vi "auton safty.vi"(11 "Updated Drive Metrics in":T1) -> (3 "Updated Drive Metrics out":T1)   [LabVIEW 2014]
uses:
  Lightning base/Drive Train Metrics.ctl
  Lightning base/CmdFlag.ctl
  Robot Global Data.vi
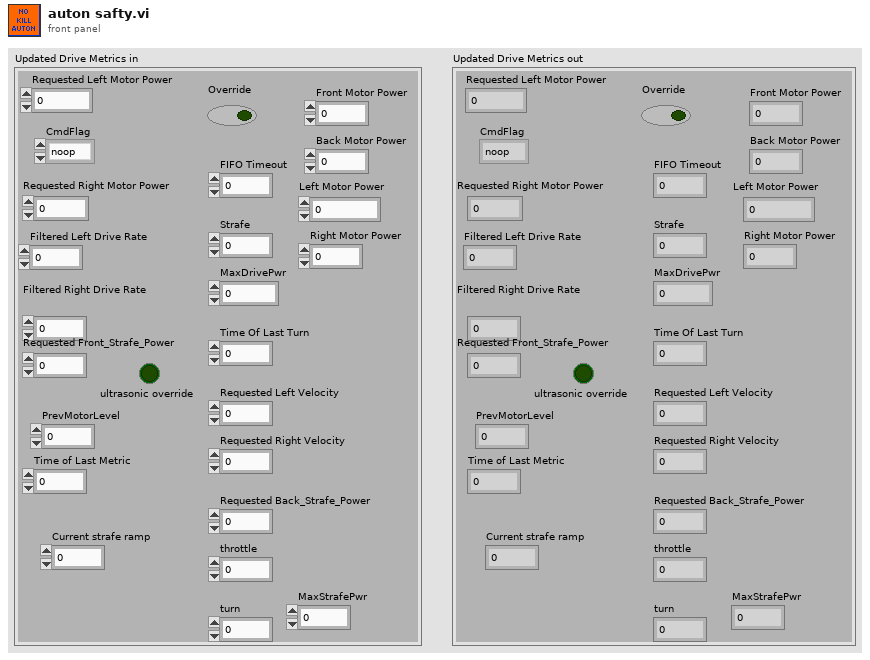
[diagram p1: front panel]
types:
  T1 = typedef "Drive Train Metrics.ctl" = cluster{"CmdFlag":T2, "Requested Right Motor Power":dbl, "Requested Left Motor Power":dbl, "Filtered Left Drive Rate":dbl, "Filtered Right Drive Rate":dbl, "Time of Last Metric":u32, "FIFO Timeout":i32, "Requested Left Velocity":dbl, "Requested Right Velocity":dbl, "throttle":dbl, "turn":dbl, "MaxDrivePwr":dbl, "Strafe":dbl, "Override":bool, "Time Of Last Turn":dbl, "Requested Front_Strafe_Power":dbl, "Requested Back_Strafe_Power":dbl, "MaxStrafePwr":dbl, "PrevMotorLevel":u8, "ultrasonic override":bool, "Left Motor Power":dbl, "Right Motor Power":dbl, "Front Motor Power":dbl, "Back Motor Power":dbl, "Current strafe ramp":dbl}
  T2 = typedef "CmdFlag.ctl" = enum16{"noop", "logflag", "suspend", "resume"}
  T3 = typedef "WPI_DriverStationRobotMode2.ctl" = enum16{"Autonomous Disabled", "Autonomous Enabled", "Teleop Disabled", "Teleop Enabled", "Disconnected", "Finish", "Test Disabled", "Test Enabled", "Emergency Stopped"}
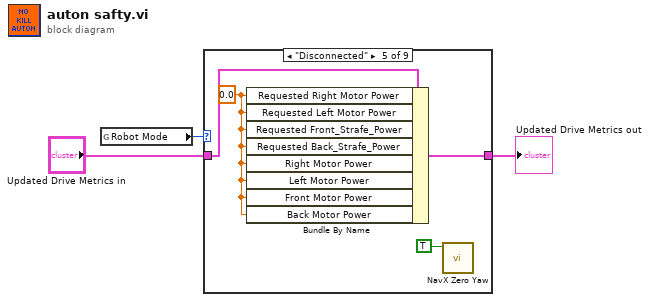
[diagram p0: block diagram]
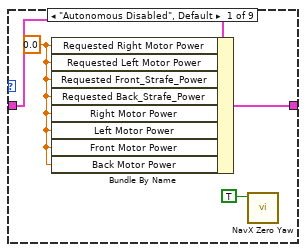
[diagram p2: hidden frame]
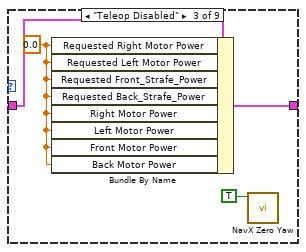
[diagram p4: hidden frame]
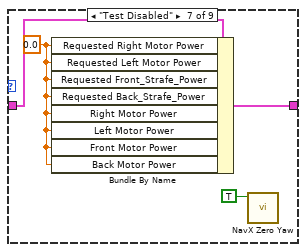
[diagram p7: hidden frame]
diagram:
  n1 = global read "Robot Global Data.vi" "Robot Mode"() -> (w3:T3)
  n2 = case shown="\"Disconnected\"" w3 {
    tunnel: "Updated Drive Metrics in" -> [w7 w8 w11 w13 w15 w18 w21 w23 w24]
    tunnel: [w5 w8 w10 w13 w14 w18 w20 w23 w24] -> w2
    frame "Autonomous Disabled", Default {
      w6 = 0.0 ("Requested Right Motor Power")
      n3 = Bundle By Name(cluster=w7, "Requested Right Motor Power"=w6, "Requested Left Motor Power"=w6, "Requested Front_Strafe_Power"=w6, "Requested Back_Strafe_Power"=w6, "Right Motor Power"=w6, "Left Motor Power"=w6, "Front Motor Power"=w6, "Back Motor Power"=w6) -> (w5:T1)
      n4 = call "NavX Zero Yaw.vi"("Reset NavX Yaw"=TRUE) -> ()  [unwired: 11 in]
    }
    frame "Autonomous Enabled" {
    }
    frame "Teleop Disabled" {
      w12 = 0.0 ("Requested Right Motor Power")
      n5 = Bundle By Name(cluster=w11, "Requested Right Motor Power"=w12, "Requested Left Motor Power"=w12, "Requested Front_Strafe_Power"=w12, "Requested Back_Strafe_Power"=w12, "Right Motor Power"=w12, "Left Motor Power"=w12, "Front Motor Power"=w12, "Back Motor Power"=w12) -> (w10:T1)
      n6 = call "NavX Zero Yaw.vi"("Reset NavX Yaw"=TRUE) -> ()  [unwired: 11 in]
    }
    frame "Teleop Enabled" {
    }
    frame "Disconnected" {
      w17 = 0.0 ("Requested Right Motor Power")
      n7 = Bundle By Name(cluster=w15, "Requested Right Motor Power"=w17, "Requested Left Motor Power"=w17, "Requested Front_Strafe_Power"=w17, "Requested Back_Strafe_Power"=w17, "Right Motor Power"=w17, "Left Motor Power"=w17, "Front Motor Power"=w17, "Back Motor Power"=w17) -> (w14:T1)
      n8 = call "NavX Zero Yaw.vi"("Reset NavX Yaw"=TRUE) -> ()  [unwired: 11 in]
    }
    frame "Finish" {
    }
    frame "Test Disabled" {
      w22 = 0.0 ("Requested Right Motor Power")
      n9 = Bundle By Name(cluster=w21, "Requested Right Motor Power"=w22, "Requested Left Motor Power"=w22, "Requested Front_Strafe_Power"=w22, "Requested Back_Strafe_Power"=w22, "Right Motor Power"=w22, "Left Motor Power"=w22, "Front Motor Power"=w22, "Back Motor Power"=w22) -> (w20:T1)
      n10 = call "NavX Zero Yaw.vi"("Reset NavX Yaw"=TRUE) -> ()  [unwired: 11 in]
    }
    frame "Test Enabled" {
    }
    frame "Emergency Stopped" {
    }
  }
  "Updated Drive Metrics out" <- w2
